vi "Make sound using waveform.vi"() -> ()   [LabVIEW 2015]
uses:
  <vilib>/Analysis/NI_AALBase.lvlib
panel:
  in  "Boolean 6":bool
  in  "Boolean 5":bool
  in  "Boolean 4":bool
  in  "Boolean 3":bool
  in  "Boolean 2":bool
  in  "Boolean":bool
  out "Waveform Graph":waveform(dbl)(graph)
  in  "duration":dbl
  # "Make sound using waveform"
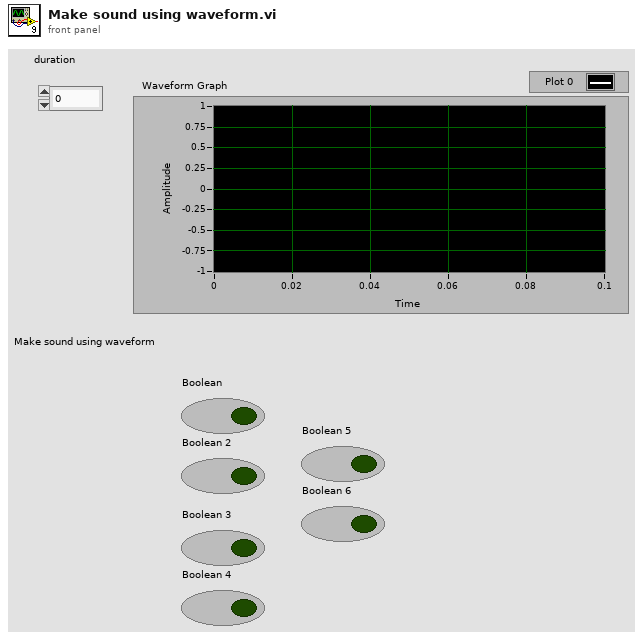
[diagram p1: front panel]
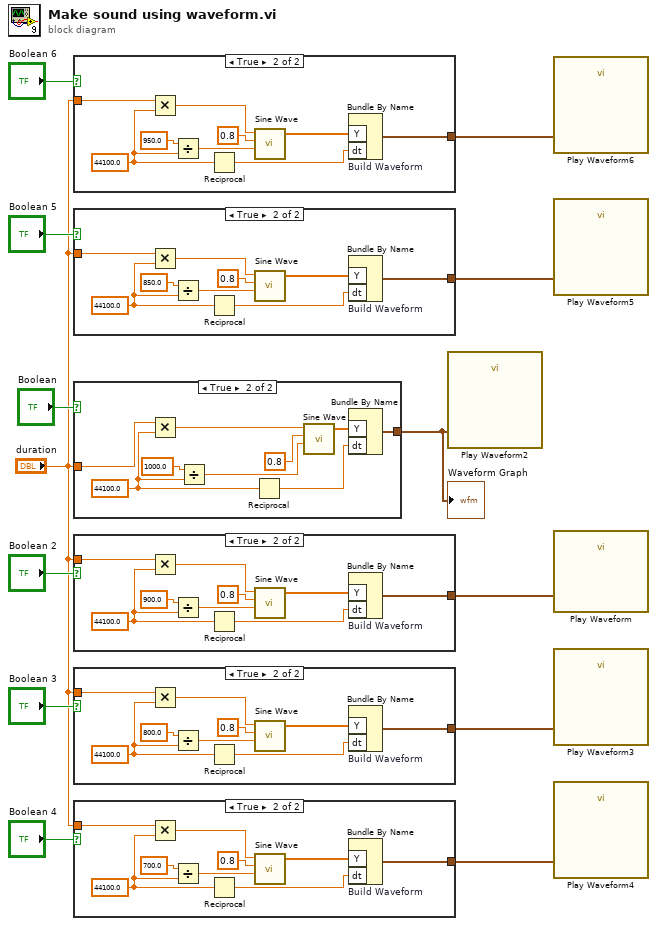
[diagram p0: block diagram]
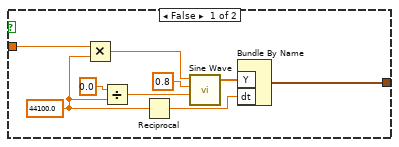
[diagram p2: hidden frame]
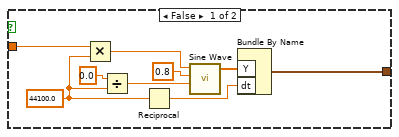
[diagram p3: hidden frame]
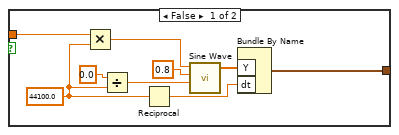
[diagram p4: hidden frame]
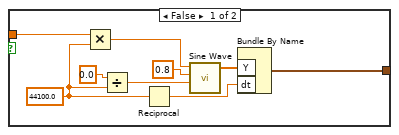
[diagram p5: hidden frame]
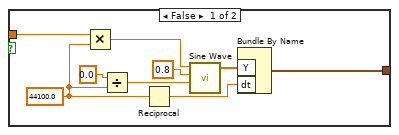
[diagram p6: hidden frame]
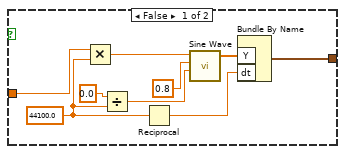
[diagram p7: hidden frame]
diagram:
  n1 = case shown="True" "Boolean 6" {
    tunnel: "duration" -> [w15 w25]
    tunnel: [w14 w24] -> w3
    frame False {
      w20 = 44100.0 ("fs(HZ) 3")
      n2 = Multiply(x=w15, y=w20) -> (x*y=w17:dbl)
      n3 = Divide(x=0.0 ("f(HZ) 2"), y=w20) -> (x/y=w18:dbl)
      n4 = Reciprocal(x=w20) -> (1/x=w21:dbl)
      n5 = call <vilib>:"Sine Wave.vi"("samples"=w17, "amplitude"=0.8, "frequency"=w18) -> ("sine wave"=w22:dbl[])  [unwired: 2 in, 2 out]
      n6 = Bundle By Name("Y"=w22, "dt"=w21) -> (w14:waveform(dbl))  [unwired: 1 in]
    }
    frame True {
      w29 = 44100.0 ("fs(HZ) 3")
      n7 = Multiply(x=w25, y=w29) -> (x*y=w26:dbl)
      n8 = Divide(x=950.0 ("f(HZ) 2"), y=w29) -> (x/y=w27:dbl)
      n9 = Reciprocal(x=w29) -> (1/x=w30:dbl)
      n10 = call <vilib>:"Sine Wave.vi"("samples"=w26, "amplitude"=0.8, "frequency"=w27) -> ("sine wave"=w31:dbl[])  [unwired: 2 in, 2 out]
      n11 = Bundle By Name "Build Waveform"("Y"=w31, "dt"=w30) -> (w24:waveform(dbl))  [unwired: 1 in]
    }
  }
  n12 = case shown="True" "Boolean 5" {
    tunnel: "duration" -> [w33 w43]
    tunnel: [w32 w42] -> w5
    frame False {
      w38 = 44100.0 ("fs(HZ) 3")
      n13 = Multiply(x=w33, y=w38) -> (x*y=w35:dbl)
      n14 = Divide(x=0.0 ("f(HZ) 2"), y=w38) -> (x/y=w36:dbl)
      n15 = Reciprocal(x=w38) -> (1/x=w39:dbl)
      n16 = call <vilib>:"Sine Wave.vi"("samples"=w35, "amplitude"=0.8, "frequency"=w36) -> ("sine wave"=w40:dbl[])  [unwired: 2 in, 2 out]
      n17 = Bundle By Name("Y"=w40, "dt"=w39) -> (w32:waveform(dbl))  [unwired: 1 in]
    }
    frame True {
      w47 = 44100.0 ("fs(HZ) 3")
      n18 = Multiply(x=w43, y=w47) -> (x*y=w44:dbl)
      n19 = Divide(x=850.0 ("f(HZ) 2"), y=w47) -> (x/y=w45:dbl)
      n20 = Reciprocal(x=w47) -> (1/x=w48:dbl)
      n21 = call <vilib>:"Sine Wave.vi"("samples"=w44, "amplitude"=0.8, "frequency"=w45) -> ("sine wave"=w49:dbl[])  [unwired: 2 in, 2 out]
      n22 = Bundle By Name "Build Waveform"("Y"=w49, "dt"=w48) -> (w42:waveform(dbl))  [unwired: 1 in]
    }
  }
  n23 = case shown="True" "Boolean" {
    tunnel: "duration" -> [w51 w61]
    tunnel: [w50 w60] -> w1
    frame False {
      w56 = 44100.0 ("fs(HZ) 3")
      n24 = Multiply(x=w51, y=w56) -> (x*y=w53:dbl)
      n25 = Divide(x=0.0 ("f(HZ) 2"), y=w56) -> (x/y=w54:dbl)
      n26 = Reciprocal(x=w56) -> (1/x=w57:dbl)
      n27 = call <vilib>:"Sine Wave.vi"("samples"=w53, "amplitude"=0.8, "frequency"=w54) -> ("sine wave"=w58:dbl[])  [unwired: 2 in, 2 out]
      n28 = Bundle By Name("Y"=w58, "dt"=w57) -> (w50:waveform(dbl))  [unwired: 1 in]
    }
    frame True {
      w65 = 44100.0 ("fs(HZ) 3")
      n29 = Multiply(x=w61, y=w65) -> (x*y=w62:dbl)
      n30 = Divide(x=1000.0 ("f(HZ) 2"), y=w65) -> (x/y=w63:dbl)
      n31 = Reciprocal(x=w65) -> (1/x=w66:dbl)
      n32 = call <vilib>:"Sine Wave.vi"("samples"=w62, "amplitude"=0.8, "frequency"=w63) -> ("sine wave"=w67:dbl[])  [unwired: 2 in, 2 out]
      n33 = Bundle By Name("Y"=w67, "dt"=w66) -> (w60:waveform(dbl))  [unwired: 1 in]
    }
  }
  "Waveform Graph" <- w1
  n34 = case shown="True" "Boolean 2" {
    tunnel: "duration" -> [w69 w79]
    tunnel: [w68 w78] -> w11
    frame False {
      w74 = 44100.0 ("fs(HZ) 3")
      n35 = Multiply(x=w69, y=w74) -> (x*y=w71:dbl)
      n36 = Divide(x=0.0 ("f(HZ) 2"), y=w74) -> (x/y=w72:dbl)
      n37 = Reciprocal(x=w74) -> (1/x=w75:dbl)
      n38 = call <vilib>:"Sine Wave.vi"("samples"=w71, "amplitude"=0.8, "frequency"=w72) -> ("sine wave"=w76:dbl[])  [unwired: 2 in, 2 out]
      n39 = Bundle By Name("Y"=w76, "dt"=w75) -> (w68:waveform(dbl))  [unwired: 1 in]
    }
    frame True {
      w83 = 44100.0 ("fs(HZ) 3")
      n40 = Multiply(x=w79, y=w83) -> (x*y=w80:dbl)
      n41 = Divide(x=900.0 ("f(HZ) 2"), y=w83) -> (x/y=w81:dbl)
      n42 = Reciprocal(x=w83) -> (1/x=w84:dbl)
      n43 = call <vilib>:"Sine Wave.vi"("samples"=w80, "amplitude"=0.8, "frequency"=w81) -> ("sine wave"=w85:dbl[])  [unwired: 2 in, 2 out]
      n44 = Bundle By Name "Build Waveform"("Y"=w85, "dt"=w84) -> (w78:waveform(dbl))  [unwired: 1 in]
    }
  }
  n45 = case shown="True" "Boolean 3" {
    tunnel: "duration" -> [w87 w97]
    tunnel: [w86 w96] -> w9
    frame False {
      w92 = 44100.0 ("fs(HZ) 3")
      n46 = Multiply(x=w87, y=w92) -> (x*y=w89:dbl)
      n47 = Divide(x=0.0 ("f(HZ) 2"), y=w92) -> (x/y=w90:dbl)
      n48 = Reciprocal(x=w92) -> (1/x=w93:dbl)
      n49 = call <vilib>:"Sine Wave.vi"("samples"=w89, "amplitude"=0.8, "frequency"=w90) -> ("sine wave"=w94:dbl[])  [unwired: 2 in, 2 out]
      n50 = Bundle By Name("Y"=w94, "dt"=w93) -> (w86:waveform(dbl))  [unwired: 1 in]
    }
    frame True {
      w101 = 44100.0 ("fs(HZ) 3")
      n51 = Multiply(x=w97, y=w101) -> (x*y=w98:dbl)
      n52 = Divide(x=800.0 ("f(HZ) 2"), y=w101) -> (x/y=w99:dbl)
      n53 = Reciprocal(x=w101) -> (1/x=w102:dbl)
      n54 = call <vilib>:"Sine Wave.vi"("samples"=w98, "amplitude"=0.8, "frequency"=w99) -> ("sine wave"=w103:dbl[])  [unwired: 2 in, 2 out]
      n55 = Bundle By Name "Build Waveform"("Y"=w103, "dt"=w102) -> (w96:waveform(dbl))  [unwired: 1 in]
    }
  }
  n56 = case shown="True" "Boolean 4" {
    tunnel: "duration" -> [w105 w115]
    tunnel: [w104 w114] -> w7
    frame False {
      w110 = 44100.0 ("fs(HZ) 3")
      n57 = Multiply(x=w105, y=w110) -> (x*y=w107:dbl)
      n58 = Divide(x=0.0 ("f(HZ) 2"), y=w110) -> (x/y=w108:dbl)
      n59 = Reciprocal(x=w110) -> (1/x=w111:dbl)
      n60 = call <vilib>:"Sine Wave.vi"("samples"=w107, "amplitude"=0.8, "frequency"=w108) -> ("sine wave"=w112:dbl[])  [unwired: 2 in, 2 out]
      n61 = Bundle By Name("Y"=w112, "dt"=w111) -> (w104:waveform(dbl))  [unwired: 1 in]
    }
    frame True {
      w119 = 44100.0 ("fs(HZ) 3")
      n62 = Multiply(x=w115, y=w119) -> (x*y=w116:dbl)
      n63 = Divide(x=700.0 ("f(HZ) 2"), y=w119) -> (x/y=w117:dbl)
      n64 = Reciprocal(x=w119) -> (1/x=w120:dbl)
      n65 = call <vilib>:"Sine Wave.vi"("samples"=w116, "amplitude"=0.8, "frequency"=w117) -> ("sine wave"=w121:dbl[])  [unwired: 2 in, 2 out]
      n66 = Bundle By Name "Build Waveform"("Y"=w121, "dt"=w120) -> (w114:waveform(dbl))  [unwired: 1 in]
    }
  }
  n67 = call "Play Waveform2"("Data"=w1) -> ()  [unwired: 18 in, 1 out]
  n68 = call "Play Waveform6"("Data"=w3) -> ()  [unwired: 18 in, 1 out]
  n69 = call "Play Waveform5"("Data"=w5) -> ()  [unwired: 18 in, 1 out]
  n70 = call "Play Waveform"("Data"=w11) -> ()  [unwired: 18 in, 1 out]
  n71 = call "Play Waveform3"("Data"=w9) -> ()  [unwired: 18 in, 1 out]
  n72 = call "Play Waveform4"("Data"=w7) -> ()  [unwired: 18 in, 1 out]
